vi "Configure Parameter to Measure.vi"(8 "error in (no error)":errorcluster, 10 "Sparameters (string)":string[](array[string]), 11 "VNA-ENA in":refnum<class "VNA-ENA.lvclass">) -> (0 "error out":errorcluster, 3 "VNA-ENA out":refnum<class "VNA-ENA.lvclass">)   [LabVIEW 2020, in "VNA-ENA.lvclass"]
uses:
  VNA-ENA.lvclass
  C:/Sandbox/RF Bench/Source Code/WiSpry Test Framework/Instruments/Instrument.lvclass
  Instrument.lvclass/Instrument.ctl
  Instrument.lvclass
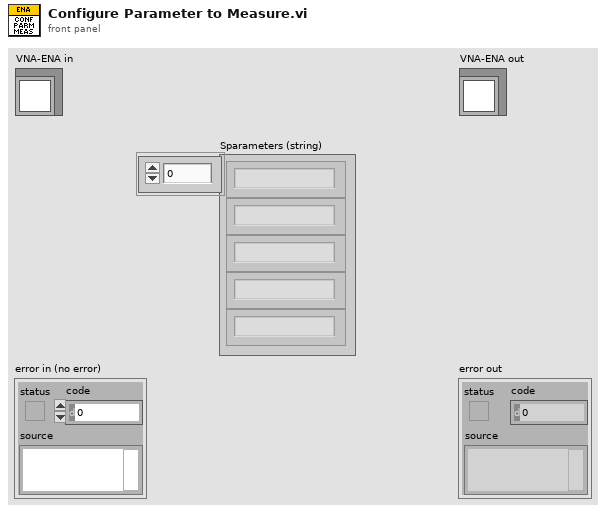
[diagram p1: front panel]
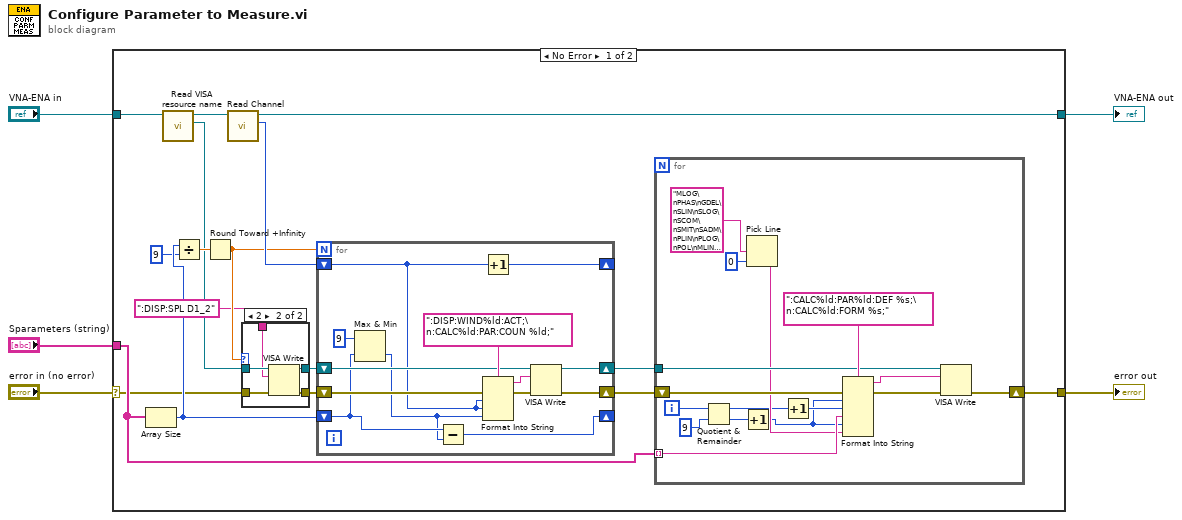
[diagram p0: block diagram]
diagram:
  n1 = case shown="No Error" "error in (no error)" {
    selector: "error in (no error)" -> [w11 w60]
    tunnel: [w19 w60] -> w4
    tunnel: [w21 w59] -> w3
    tunnel: "VNA-ENA in" -> [w22 w59]
    tunnel: "Sparameters (string)" -> [w17 _]
    frame No Error {
      n2 = Array Size(array=w17) -> (size(s)=w14:i32)
      n3 = call "Read VISA resource name.vi"("Instrument in"=w22) -> ("VISA resource name"=w9:refnum<visa-resource-name>, "Instrument out"=w20:refnum<class "VNA-ENA.lvclass">)  [unwired: 9 in]
      n4 = Divide(x=w14, y=9) -> (x/y=w12:dbl)
      n5 = Round Toward +Infinity(x=w12) -> (ceil(x): smallest int >= x=w7:dbl)
      n6 = call-dynamic "Read Channel.vi"("Vector Network Analyzer in"=w20) -> ("Channel"=w18:i32, "Vector Network Analyzer out"=w21:refnum<class "VNA-ENA.lvclass">)  [unwired: 9 in]
      n7 = case shown="2" w7 {
        tunnel: w11 -> [w24 w29]
        tunnel: [w23 w28] -> w10
        tunnel: w9 -> [w23 w27]
        tunnel: [w24 w26] -> w8
        tunnel: ":DISP:SPL D1_2" ("format string") -> [_ w25]
        frame 1, Default {
        }
        frame 2 {
          n8 = VISA Write(VISA resource name=w27, write buffer=w25, error in (no error)=w29) -> (VISA resource name out=w28:refnum<visa-resource-name>, error out=w26:errorcluster)  [unwired: 1 out]
        }
      }
      n9 = for {
        N: w7 -> [_]
        shift-right: [w36] -> w15
        shift-left: w8 -> [w41]
        shift-right: [w37] -> w16
        shift-left: w10 -> [w38]
        shift-right: [w32] -> _
        shift-left: w14 -> [w34]
        shift-right: [w30] -> _
        shift-left: w18 -> [w31]
        n10 = Max & Min(x=9, y=w34) -> (min(x,y)=w33:i32)  [unwired: 1 out]
        n11 = Subtract(x=w34, y=w33) -> (x-y=w32:i32)
        n12 = Increment(x=w31) -> (x+1=w30:i32)
        n13 = Format Into String(format string=":DISP:WIND%ld:ACT;\n:CALC%ld:PAR:COUN %ld;", error in=w41, w31, w31, w33) -> (resulting string=w39:string, error out=w40:errorcluster)  [unwired: 1 in]
        n14 = VISA Write(VISA resource name=w38, write buffer=w39, error in (no error)=w40) -> (VISA resource name out=w37:refnum<visa-resource-name>, error out=w36:errorcluster)  [unwired: 1 out]
      }
      n15 = for {
        tunnel: w17 -> [w51] mode=indexing
        tunnel: w16 -> [w54]
        shift-right: [w57] -> w19
        shift-left: w15 -> [w55]
        i -> [w47]
        n16 = Quotient & Remainder(x=w47, y=9) -> (x-y*floor(x/y)=w43:i32, floor(x/y)=w44:i32)
        n17 = Increment(x=w44) -> (x+1=w45:i32)
        n18 = Pick Line(multi-line string="MLOG\nPHAS\nGDEL\nSLIN\nSLOG\nSCOM\nSMIT\nSADM\nPLIN\nPLOG\nPOL\nMLIN\nSWR\nREAL\nIMAG\nUPH\nPPH" ("string (\"\")"), line index=0) -> (output string=w48:string)  [unwired: 1 in]
        n19 = Increment(x=w43) -> (x+1=w53:i32)
        n20 = Format Into String(format string=":CALC%ld:PAR%ld:DEF %s;\n:CALC%ld:FORM %s;", error in=w55, w45, w53, w51, w45, w48) -> (resulting string=w52:string, error out=w56:errorcluster)  [unwired: 1 in]
        n21 = VISA Write(VISA resource name=w54, write buffer=w52, error in (no error)=w56) -> (error out=w57:errorcluster)  [unwired: 2 out]
      }
    }
    frame Error {
    }
  }
  "error out" <- w4
  "VNA-ENA out" <- w3
